vi "FailureDescription.vi"(8 "error in (no error)":errorcluster, 10 "Actual":variant, 11 "Constraint in":refnum<class "Constraint.lvclass">) -> (0 "error out":errorcluster, 2 "Failure Description":string, 3 "Constraint out":refnum<class "Constraint.lvclass">)   [LabVIEW 2017, in "Transparent Assertions.lvlib" / "Constraint.lvclass"]
doc: "Return the second part of the scentence \"Failed asserting that ...\""
uses:
  Constraint.lvclass
  To JSON.vi/c34f3794-71bb-4fc1-98c1-2c7c55f09150.vi
  <vilib>/PNR/JSONtext Object Serialization/Generic Object Serializer/Generic Object Serializer.lvclass
  C:/Program Files/National Instruments/LabVIEW 2017/vi.lib/JDP Science/JSONtext/LVClass Serializer/JSONtext LVClass Serializer.lvclass
  <vilib>/JDP Science/JSONtext/Variant to JSON Text.vi
  Transparent Assertions.lvlib
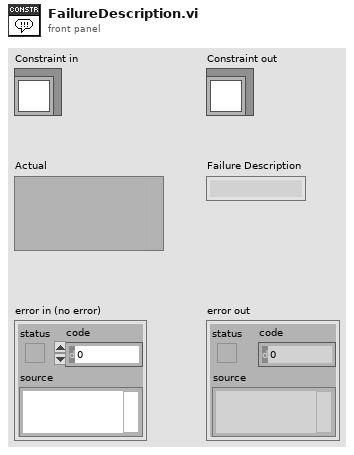
[diagram p1: front panel]
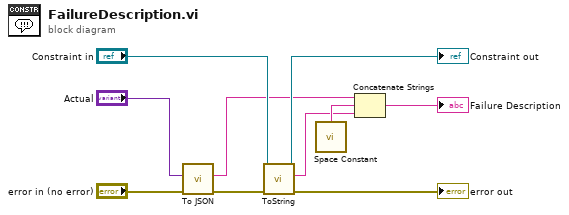
[diagram p0: block diagram]
diagram:
  n1 = call "To JSON.vi"("error in (no error)"="error in (no error)", "Anything"="Actual") -> ("error out"=w1:errorcluster, "JSON"=w3:string)  [unwired: 8 in]
  n2 = call-dynamic "ToString.vi"("error in (no error)"=w1, "Constraint in"="Constraint in") -> ("error out"=→"error out":errorcluster, "String"=w5:string, "Constraint out"=→"Constraint out":refnum<class "Constraint.lvclass">)  [unwired: 7 in]
  n3 = call <vilib>:"Space Constant.vi"() -> ("String"=w6:string)
  n4 = Concatenate Strings(w3, w6, w5) -> (→"Failure Description":string)
